vi "U32_to_hex.vi"(9 "y 3":u32=300) -> (2 "string 5":string)   [LabVIEW 2021]
panel:
  out "x-y*floor(x/y) 9":u32=2
  out "appended array 3":u32[](array[numeric])
  out "x-y*floor(x/y) 8":u32=2
  out "x-y*floor(x/y) 6":u32=2
  out "x-y*floor(x/y) 7":u32=12
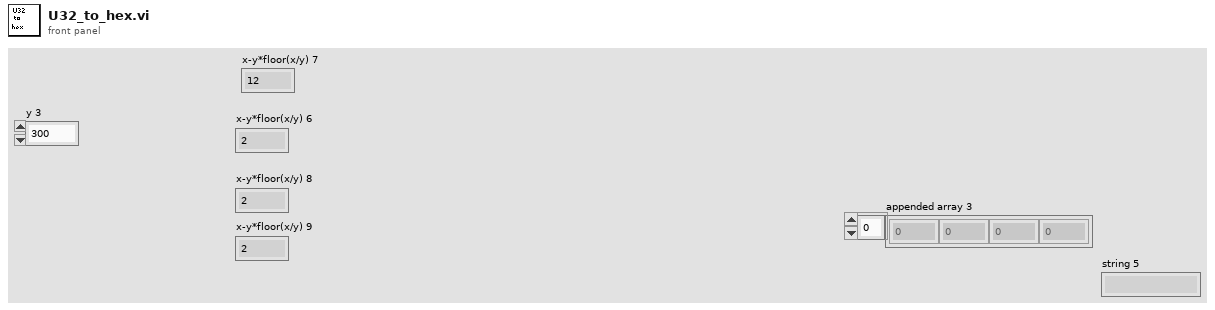
[diagram p1: front panel]
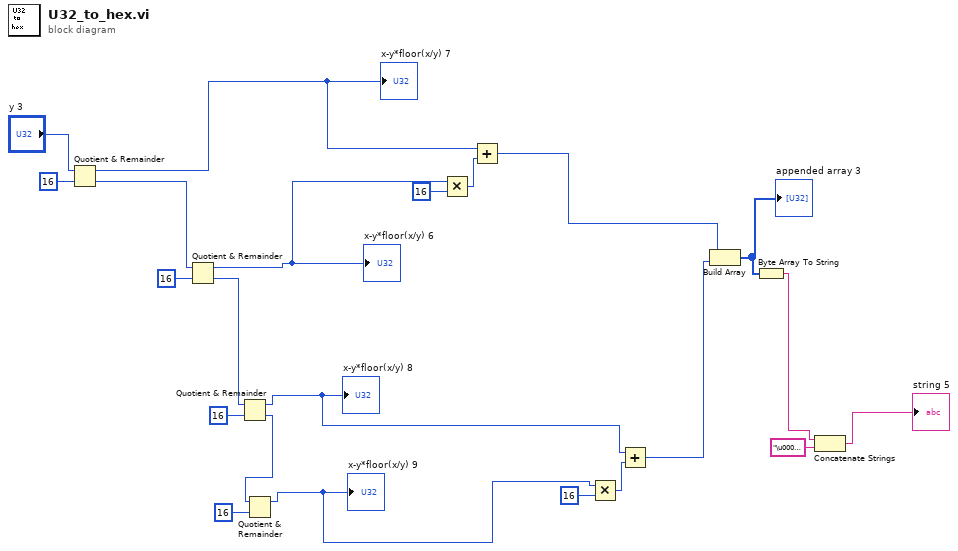
[diagram p0: block diagram]
diagram:
  n1 = Quotient & Remainder(x="y 3", y=u32 16) -> (x-y*floor(x/y)=w11:u32, floor(x/y)=w22:u32)
  "x-y*floor(x/y) 7" <- w11
  n2 = Quotient & Remainder(x=w22, y=u32 16) -> (x-y*floor(x/y)=w14:u32, floor(x/y)=w17:u32)
  "x-y*floor(x/y) 6" <- w14
  n3 = Quotient & Remainder(x=w17, y=u32 16) -> (x-y*floor(x/y)=w8:u32, floor(x/y)=w15:u32)
  "x-y*floor(x/y) 8" <- w8
  n4 = Quotient & Remainder(x=w15, y=u32 16) -> (x-y*floor(x/y)=w7:u32)  [unwired: 1 out]
  "x-y*floor(x/y) 9" <- w7
  n5 = Multiply(x=w14, y=u32 16) -> (x*y=w12:u32)
  n6 = Add(x=w11, y=w12) -> (x+y=w2:u32)
  n7 = Multiply(x=w7, y=u32 16) -> (x*y=w10:u32)
  n8 = Add(x=w8, y=w10) -> (x+y=w1:u32)
  n9 = Build Array(w2, w1) -> (w6:u32[])
  "appended array 3" <- w6
  n10 = Byte Array To String(unsigned byte array=w6) -> (string=w4:string)
  n11 = Concatenate Strings(w4, "\u0000\u0000" ("string")) -> (→"string 5":string)
